vi "LEDS_Spotlight Control.vi"(0 "Name":string, 1 "Button":bool) -> (9 "Relay State":T1)   [LabVIEW 2011]
uses:
  <vilib>/Rock Robotics/WPI/Relay/WPI_RelayValue.ctl
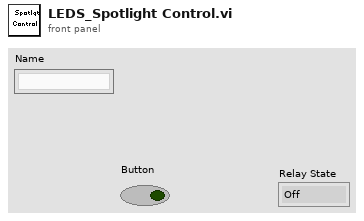
[diagram p1: front panel]
types:
  T1 = typedef "WPI_RelayValue.ctl" = enum16{"Off", "On", "Forward", "Reverse"}
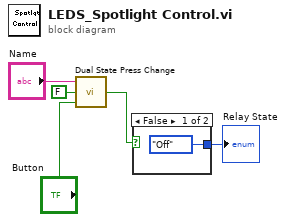
[diagram p0: block diagram]
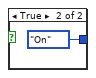
[diagram p2: hidden frame]
diagram:
  n1 = call "Dual State Press Change.vi"("Enable/Disable"="Button", "Initial"=FALSE, "Value Name"="Name") -> ("Enabled"=w4:bool)
  n2 = case shown="False" w4 {
    tunnel: [WPI_RelayValue."Off" ("RelayValue") WPI_RelayValue."On" ("RelayValue")] -> w5
    frame False {
    }
    frame True {
    }
  }
  "Relay State" <- w5
